vi "WriteSGL.vi"(10 "Data":sgl, 11 "Address":u32) -> ()   [LabVIEW 2016]
uses:
  <vilib>/rvi/Memory/Memory_Emulation/nirvimemoryFastEmulation.vi
  <vilib>/rvi/Memory/Memory_Emulation/nirvimemoryEmulation.vi
  <vilib>/rvi/Emulation/niFpgaEmulationIsFPGAContextNoSignature.vi
  <vilib>/rvi/DataTransferAndStorage/Container/Common/niFpgaContainerGetUniqueNameForEmu.vi
  <vilib>/rvi/Emulation/niFpgaProcessEmulError.vi
  <vilib>/rvi/Emulation/niFpgaSctlEmulationGetInTimedLoop.vi
  <vilib>/rvi/errors/nirviReportUnexpectedCaseInternalError (U32).vi
  <vilib>/rvi/DataTransferAndStorage/Container/Common/niFpgaContainerExecOnDevCompGetState.vi
  <vilib>/rvi/Memory/Memory_Emulation/niFpgaMemoryEmulationCacheClearOnFirstRun.vi
  <vilib>/rvi/Memory/Memory_Emulation/nirvimemoryEmulationManagerCache_MakeExclusive.vi
  <vilib>/rvi/Memory/Memory_Emulation/niFpgaMemoryEmulationValidateCache.vi
  <vilib>/rvi/Memory/Memory_Emulation/nirvimemoryEmulationManagerCache_InsertValue.vi
  <vilib>/Utility/error.llb/Clear Errors.vi
  <vilib>/rvi/Memory/Memory_Emulation/nirvimemoryEmulationManagerCache_ReleaseExclusive.vi
  <vilib>/rvi/Memory/Memory_Emulation/nirvimemoryEmulationManagerCache_GetValue.vi
  <vilib>/rvi/Memory/Memory_Emulation/nirvimemoryEmulationManagerCache_SetValue.vi
  <vilib>/rvi/Emulation/niFpgaSctlEmulationResourceMgr.vi
  <vilib>/rvi/DataTransferAndStorage/Container/XNode/niFpgaContainer.xnode
  <vilib>/rvi/Memory/Memory_Emulation/niFpgaMemoryEmulationRefIn.vi
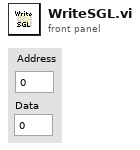
[diagram p1: front panel]
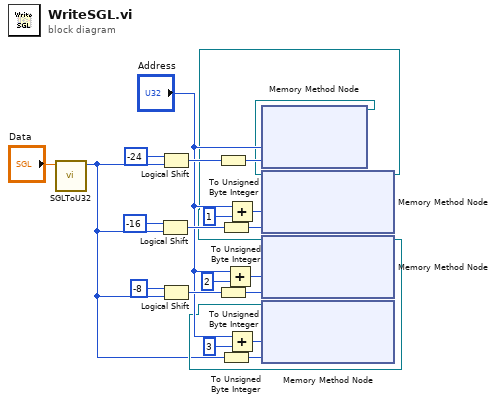
[diagram p0: block diagram]
diagram:
  n1 = call "SGLToU32.vi"("SGL"="Data") -> ("U32"=w1:u32)  [unwired: 10 in]
  n2 = Logical Shift(y=i16 -16, x=w1) -> (x << y=w7:u32)
  n3 = Logical Shift(y=i16 -24, x=w1) -> (x << y=w18:u32)
  n4 = Logical Shift(y=i16 -8, x=w1) -> (x << y=w15:u32)
  n5 = To Unsigned Byte Integer(number=w18) -> (unsigned 8bit integer=w19:u8)
  n6 = To Unsigned Byte Integer(number=w15) -> (unsigned 8bit integer=w14:u8)
  n7 = To Unsigned Byte Integer(number=w7) -> (unsigned 8bit integer=w17:u8)
  n8 = To Unsigned Byte Integer(number=w1) -> (unsigned 8bit integer=w16:u8)
  n9 = Add(x="Address", y=u32 2) -> (x+y=w9:u32)
  n10 = Add(x="Address", y=u32 1) -> (x+y=w22:u32)
  n11 = Add(x="Address", y=u32 3) -> (x+y=w11:u32)
  n12 = xnode ("Memory Method Node")("Address"="Address", "Data"=w19) -> ("Memory Out"=w5:refnum<k21>)  [unwired: 1 in]
  n13 = xnode ("Memory Method Node")("Address"=w22, "Data"=w17, "Memory In"=w5) -> ("Memory Out"=w4:refnum<k21>)
  n14 = xnode ("Memory Method Node")("Address"=w9, "Data"=w14, "Memory In"=w4) -> ("Memory Out"=w3:refnum<k21>)
  n15 = xnode ("Memory Method Node")("Address"=w11, "Data"=w16, "Memory In"=w3) -> ()  [unwired: 1 out]
